vi "basic - Transmit (from FIle).vi"() -> ()   [LabVIEW 2020]
doc: "Overview: Setup the board to transmit package as raw frames.\nRequirement: One AIM ARINC-664 board with installed AIM ARINC 664 BSP.\nRestrictions: None.\nInstruction:\n1. Select the Board ID (0 if you have only one board in your system) and the port number. If you want to validate between two ports in one device, you can use tx board and Rx Board\n2. Run the VI.\n3. See the result in the Indicators and press STOP to stop the VI.s\nFor detailed information about functions use, see documents in <BSP Installation folder>\\AIM GmbH\\Arinc 664 Windows BSP <version>\\Doc."
uses:
  Frame Configuration/controls/frame_file_entry.ctl
  Frame Configuration/controls/frame_record_type.ctl
  <instrlib>/AIM GmbH/_AIM 664/_controls/queue_header_generic.ctl
  <instrlib>/AIM GmbH/_AIM 664/bsp/Fdx Create Session (Tx-Generic).vi
  <instrlib>/AIM GmbH/_AIM 664/bsp/Fdx Start (Tx).vi
  <instrlib>/AIM GmbH/_AIM 664/bsp/Fdx Stop (Tx).vi
  <instrlib>/AIM GmbH/_AIM 664/AIM664LV.lvlib
panel:
  in  "from file":bool
  in  "data":T1[](array[typedef]) {"value"."Data" format="%.0x"; "value"."HeaderInfo"."NetSelect" items=["FDX_TX_FRAME_DLY_A"=0, "FDX_TX_FRAME_DLY_B"=1, "FDX_TX_FRAME_BOTH "=3, "FDX_TX_FRAME_ONLY_A"=4, "FDX_TX_FRAME_ONLY_B "=5]; "value"."HeaderInfo"."FrameStartMode" items=["FDX_TX_FRAME_START_IFG", "FDX_TX_FRAME_START_PGWT", "FDX_TX_FRAME_START_TRG"]; "value"."HeaderInfo"."PhysErrorInjection" items=["FDX_TX_FRAME_ERR_OFF"=0, "FDX_TX_FRAME_ERR_CRC"=1, "FDX_TX_FRAME_ERR_ALI"=2, "FDX_TX_FRAME_ERR_PRE"=4, "FDX_TX_FRAME_ERR_PHY"=8]; "value"."HeaderInfo"."SequenceNumberInit" items=["FDX_TX_FRAME_SEQ_INIT_AUTO"=65535]; "value"."HeaderInfo"."SequenceNumberOffset" items=["FDX_TX_FRAME_SEQ_OFFS_AUTO "=65535]; "value"."HeaderInfo"."PayloadGenerationMode" items=["FDX_TX_FRAME_PGM_USER"=0, "FDX_TX_FRAME_PGM_IP_PART"=1, "FDX_TX_FRAME_PGM_IP_FULL"=2, "FDX_TX_FRAME_PGM_IP_PART_TT"=10, "FDX_TX_FRAME_PGM_IP_FULL_TT"=20]; "value"."HeaderInfo"."PayloadBufferMode" items=["FDX_TX_FRAME_PBM_STD", "FDX_TX_FRAME_PBM_MAC", "FDX_TX_FRAME_PBM_UDP"]}
  in  "file path (use dialog)":path=path "/home/lvuser/T2_TxRxMon_HARDWARE_board0_v1.bin"
  in  "PortMap":u32
  out "Duplicated":bool
  out "TxStatus":T4={"TxStatus"=1, "Frames"=855, "TransmitMode"=0, "FramesPortB"=0}
  out "TxQueueStatus":T5={"QueueStatus"=0, "BytesReloadable"=0, "FramesSent"=854, "FramesInCycQueue"=0} {"QueueStatus" items=["FDX_QUE_EMPTY", "FDX_QUE_FILLED", "FDX_QUE_FULL", "FDX_QUE_SENT", "FDX_QUE_CYCL_RUN", "FDX_QUE_CYCL_SENT"]}
  out "TxQueueInfo":cluster{"QueueBaseAddr":u32, "QueueSizeOut":u32}={"QueueBaseAddr"=50892800, "QueueSizeOut"=4194304}
  in  "Port":u32
  in  "Board":u32
  out "current time":timestamp=timestamp(3686777794.875688 s since 1904-01-01)
  out "current irig time":T6={"SignOut"=40, "DayOut"=1, "HourOut"=1, "MinOut"=28, "SecondOut"=39, "MilliSecOut"=539, "MicroSecOut"=300, "NanoSecOut"=0, "InfoOut"=0, "Mode"=3}
  in  "stop":bool
  out "PortInitOut":T7={"PortConfig"=0, "PortUsed"=1, "GlobalMemFree"=0, "SharedMemFree"=0} {"PortConfig" items=["FDX_SINGLE", "FDX_REDUNDANT"]}
  out "error out":errorcluster
  # "ARINC 664 - Transmitting Frames"
  # "Overview: Setup the board to transmit package as raw frames.\nRequirement: One AIM ARINC-664 board with installed AIM ARINC 664 BSP.\nRestrictions: None.\nInstruction:\n1. Select the Board ID (0 if you have only one board in your system) and the port number. If you want to validate between two ports in one device, you can use tx board and Rx Board\n2. Run the VI.\n3. See the result in the Indicators and press STOP to stop the VI."
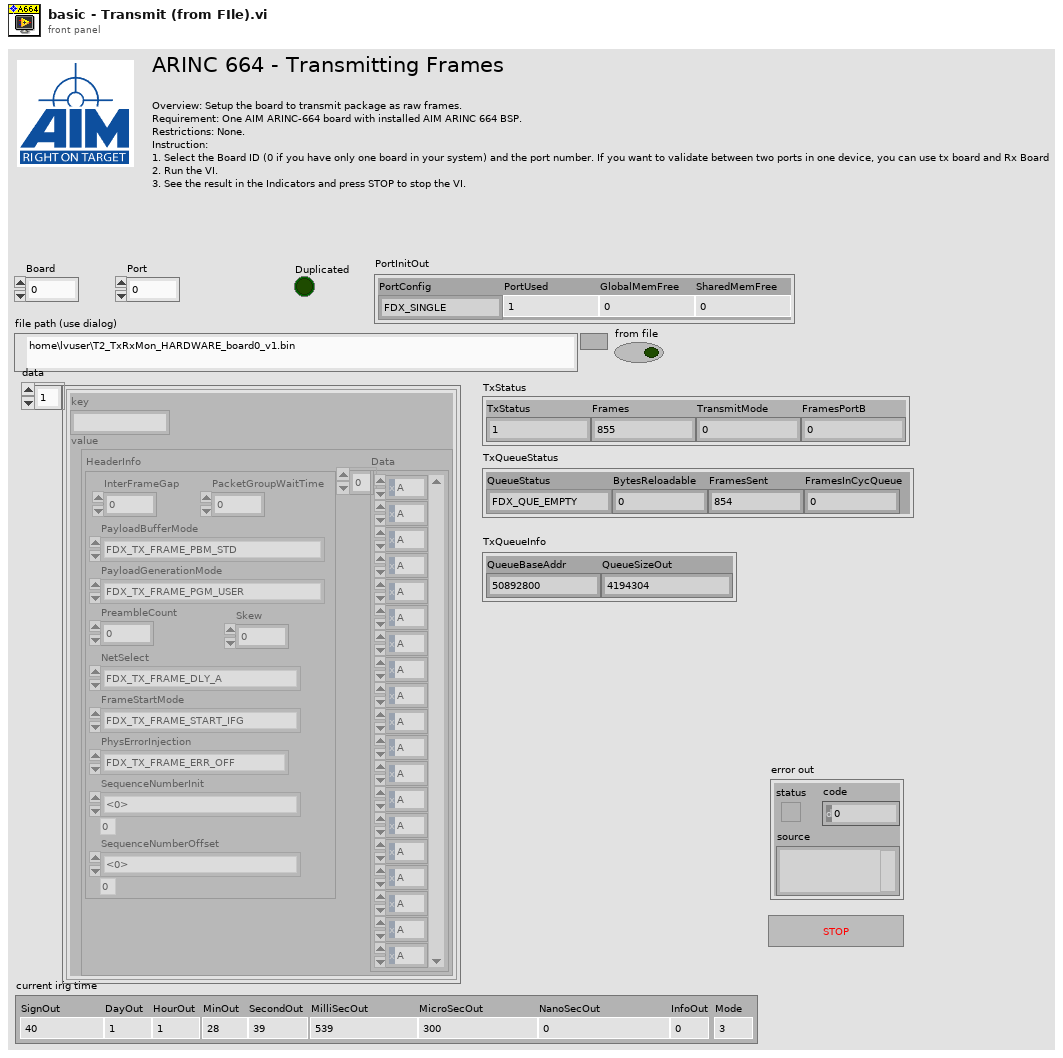
[diagram p1: front panel]
types:
  T1 = typedef "frame_file_entry.ctl" = cluster{"key":string, "value":T2}
  T2 = typedef "frame_record_type.ctl" = cluster{"HeaderInfo":T3, "Data":u8[]}
  T3 = typedef "AIM664LV.lvlib/queue_header_generic.ctl" = cluster{"InterFrameGap":u32, "PacketGroupWaitTime":u32, "PayloadBufferMode":u8, "PayloadGenerationMode":u8, "PreambleCount":u8, "Skew":u32, "NetSelect":u8, "FrameStartMode":u8, "PhysErrorInjection":u32, "SequenceNumberInit":u16, "SequenceNumberOffset":u16}
  T4 = cluster{"TxStatus":u32, "Frames":u32, "TransmitMode":u32, "FramesPortB":u32}
  T5 = cluster{"QueueStatus":i32, "BytesReloadable":u32, "FramesSent":u32, "FramesInCycQueue":u32}
  T6 = cluster{"SignOut":i32, "DayOut":u32, "HourOut":u32, "MinOut":u32, "SecondOut":u32, "MilliSecOut":u32, "MicroSecOut":u32, "NanoSecOut":u32, "InfoOut":u32, "Mode":u32}
  T7 = cluster{"PortConfig":u32, "PortUsed":u32, "GlobalMemFree":u32, "SharedMemFree":u32}
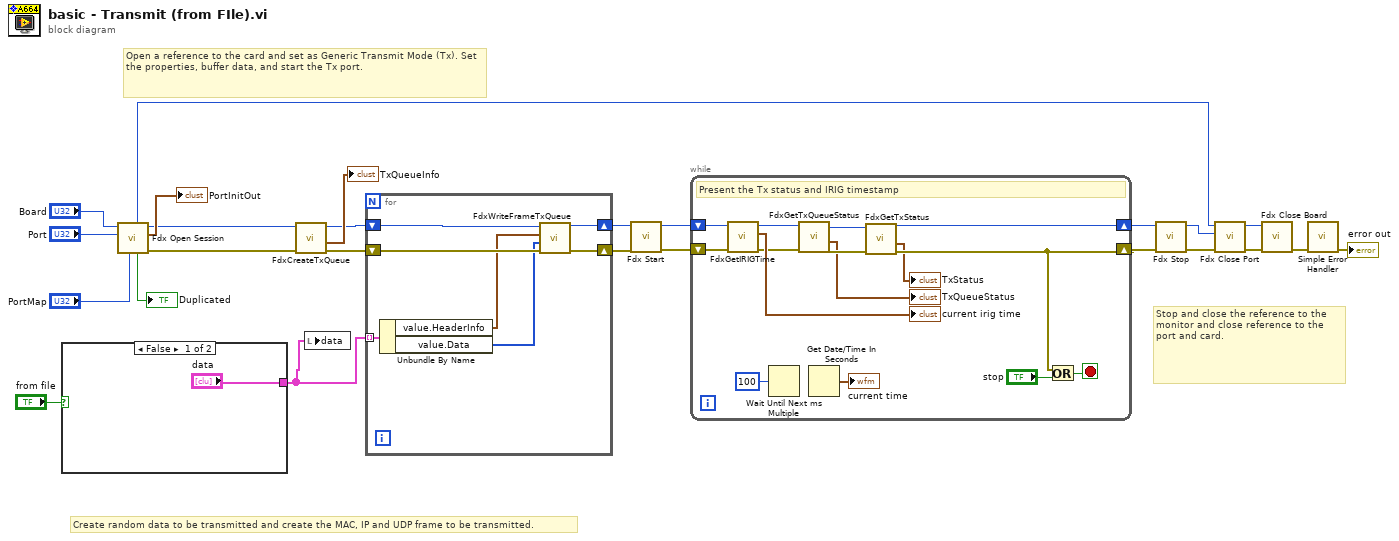
[diagram p0: block diagram]
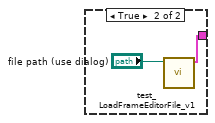
[diagram p2: hidden frame]
diagram:
  # "Stop and close the reference to the monitor and close reference to the port and card."
  # "Create random data to be transmitted and create the MAC, IP and UDP frame to be transmitted."
  # "Open a reference to the card and set as Generic Transmit Mode (Tx). Set the properties, buffer data, and start the Tx port."
  n1 = case shown="False" "from file" {
    tunnel: ["data" w27] -> w1
    frame False {
    }
    frame True {
      n2 = call "test_LoadFrameEditorFile_v1.vi"("BIN file path"="file path (use dialog)") -> ("data"=w27:T1[])  [unwired: 9 in, 1 out]
    }
  }
  n3 = call-poly <instrlib>:"Fdx Open Session.vi"("PortMap"="PortMap", "port"="Port", "board"="Board") -> ("error out"=w19:errorcluster, "PortInitOut"=→"PortInitOut":T7, "port handle out"=w20:u32, "Duplicated"=→"Duplicated":bool, "InstrumentHandle_board out"=w7:u32)  [unwired: 3 in, 1 out]
  n4 = call <instrlib>:"FdxCreateTxQueue.vi"("error in"=w19, "InstrumentHandle_port"=w20) -> ("error out"=w17:errorcluster, "TxQueueInfo"=→"TxQueueInfo":cluster{"QueueBaseAddr":u32, "QueueSizeOut":u32}, "InstrumentHandle_port"=w14:u32)  [unwired: 7 in]
  n5 = local write "data"(w1) -> ()
  n6 = for {
    shift-right: [w34] -> w16
    shift-left: w17 -> [w35]
    shift-right: [w33] -> w15
    shift-left: w14 -> [w32]
    tunnel: w1 -> [w31] mode=indexing
    n7 = Unbundle By Name(w31) -> ("value.HeaderInfo"=w30:T3, "value.Data"=w29:u8[])
    n8 = call <instrlib>:"FdxWriteFrameTxQueue.vi"("error in (no error)"=w35, "Frame in"=w29, "HeaderInfo"=w30, "InstrumentHandle_port in"=w32) -> ("error out"=w34:errorcluster, "InstrumentHandle_port out"=w33:u32)  [unwired: 6 in]
  }
  n9 = call-poly <instrlib>:"Fdx Start.vi"("error in"=w16, "InstrumentHandle_port in"=w15) -> ("error out"=w24:errorcluster, "InstrumentHandle_port out"=w23:u32)  [unwired: 8 in]
  n10 = while {
    shift-right: [w40] -> w12
    shift-left: w23 -> [w36]
    shift-right: [w41] -> w13
    shift-left: w24 -> [w37]
    stop <- w49 stop-if-true
    # "Present the Tx status and IRIG timestamp"
    n11 = call <instrlib>:"FdxGetIRIGTime.vi"("error in"=w37, "InstrumentHandle_board in"=w36) -> ("error out"=w44:errorcluster, "Curent Irig Time"=→"current irig time":T6, "InstrumentHandle_board out"=w45:u32)  [unwired: 7 in]
    n12 = Wait Until Next ms Multiple(millisecond multiple=u32 100) -> ()  [unwired: 1 out]
    n13 = call <instrlib>:"FdxGetTxQueueStatus.vi"("error in"=w44, "InstrumentHandle"=w45) -> ("error out"=w42:errorcluster, "TxQueueStatus"=→"TxQueueStatus":T5, "InstrumentHandle"=w43:u32)  [unwired: 7 in]
    n14 = Get Date/Time In Seconds() -> (seconds since 1Jan1904=→"current time":timestamp)
    n15 = call <instrlib>:"FdxGetTxStatus.vi"("error in"=w42, "InstrumentHandle_port"=w43) -> ("error out"=w41:errorcluster, "TxStatus"=→"TxStatus":T4, "InstrumentHandle_port"=w40:u32)  [unwired: 7 in]
    n16 = Or(x=w41, y="stop") -> (x .or. y?=w49:bool)
  }
  n17 = call-poly <instrlib>:"Fdx Stop.vi"("error in"=w13, "InstrumentHandle_port in"=w12) -> ("error out"=w21:errorcluster, "InstrumentHandle_port out"=w9:u32)  [unwired: 8 in]
  n18 = call <instrlib>:"Fdx Close Port.vi"("error in"=w21, "InstrumentHandle_port in"=w9, "InstrumentHandle_board in"=w7) -> ("error out"=w6:errorcluster, "InstrumentHandle_board out"=w3:u32)  [unwired: 7 in]
  n19 = call <instrlib>:"Fdx Close Board.vi"("error in"=w6, "InstrumentHandle_board in"=w3) -> ("error out"=w4:errorcluster)  [unwired: 9 in]
  n20 = call <vilib>:"Simple Error Handler.vi"("error in (no error)"=w4) -> ("error out"=→"error out":errorcluster)  [unwired: 4 in, 4 out]
